vi "Sprache aendern.vi"(8 "Fehler (Eingang, kein Fehler)":errorcluster, 10 "Zustand":T1, 11 "Cluster (Eingang)":refnum<vi>) -> (0 "error out":errorcluster caption="Fehler (Ausgang)", 3 "Controls[]":refnum<vi>[](array[refnum]))   [LabVIEW 2020, in "Funktionstasten.lvlib"]
uses:
  Funktionstasten.lvlib
  Zustaende.ctl
  Sprachverwaltung/FGV Aktion Tabelle zerlegen.ctl
  Sprachverwaltung/Sprachverwaltung.lvlib
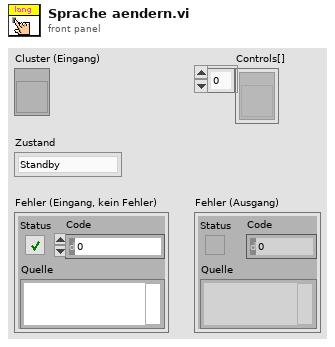
[diagram p1: front panel]
types:
  T1 = typedef "Funktionstasten.lvlib/Zustaende.ctl" = enum16{"Standby", "Pause", "Eco", "Messen", "Kalibrieren", "Spülen Filter", "Spülen Leitung", "Umgebungsluft", "0-Gas", "Cal-Gas", "CG zu PNS", "-------------", "Init 1", "Init 2", "Init 3", "Init 4", "Messen vorbereiten", "Messen durchführen", "Exit"}
  T2 = typedef "Sprachverwaltung.lvlib/FGV Aktion Tabelle zerlegen.ctl" = enum16{"laden", "vereinzeln", "speichern"}
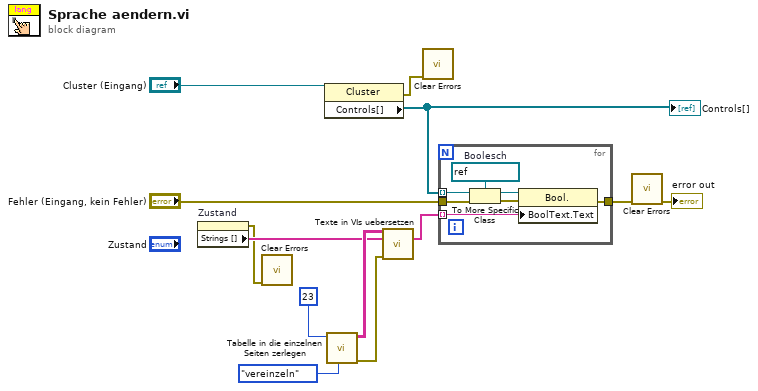
[diagram p0: block diagram]
diagram:
  n1 = property on="Zustand" class="Enum (strikt)"() -> (error out=w2:errorcluster, "Strings []"=w3:string[])  [unwired: 2 in, 1 out]
  n2 = call <vilib>:"Clear Errors.vi"("error in (no error)"=w2) -> ()  [unwired: 5 in, 2 out]
  n3 = property class="Cluster"(reference="Cluster (Eingang)") -> (error out=w6:errorcluster, "Controls[]"=w5:refnum<vi>[])  [unwired: 1 in, 1 out]
  "Controls[]" <- w5
  n4 = call "Tabelle in die einzelnen Seiten zerlegen.vi"("Aktion"=FGV_Aktion_Tabelle_zerlegen."vereinzeln", "Index (Seite)"=23) -> ("error out"=w13:errorcluster, "Sprachliste"=w10:string[][])  [unwired: 7 in, 1 out]
  n5 = call "Texte in VIs uebersetzen.vi"("Sprachliste"=w10, "String-Array zum Übersetzen"=w3, "error in (no error)"=w13) -> ("String-Array zum Übersetzen"=w11:string[])  [unwired: 8 in, 4 out]
  n6 = call <vilib>:"Clear Errors.vi"("error in (no error)"=w6) -> ()  [unwired: 5 in, 2 out]
  n7 = for {
    tunnel: w11 -> [w17] mode=indexing
    tunnel: w5 -> [w19] mode=indexing
    tunnel: "Fehler (Eingang, kein Fehler)" -> [w15]
    tunnel: [w14] -> w8
    w20 = refnum<vi> refnum  # Boolesch
    n8 = To More Specific Class(target class=w20, reference=w19, error in=w15) -> (specific class reference=w18:refnum<vi>, error out=w16:errorcluster)
    n9 = property class="Bool."(reference=w18, error in=w16, "BoolText.Text"=w17) -> (error out=w14:errorcluster)  [unwired: 1 out]
  }
  n10 = call <vilib>:"Clear Errors.vi"("error in (no error)"=w8) -> ("error out"=→"error out":errorcluster)  [unwired: 5 in, 1 out]
